vi "CosimModulator.vi"() -> ()   [LabVIEW 2017]
uses:
  FPGA/modInput.ctl
  <vilib>/Simulation/Scripting/Companion Diagram/SimConfigNode/SimParams.ctl
  <vilib>/Simulation/Scripting/Companion Diagram/SimConfigNode/_simSolvers.ctl
  <vilib>/Simulation/Implementation/Shared/SIMSCR Execution Mode.ctl
  <vilib>/Simulation/Param Hierarchy/Typedefs/SIMPH Param Control Actions.ctl
  <vilib>/Simulation/Implementation/Shared/NILVSim_ParamChanged.vi
  <vilib>/Simulation/Implementation/Shared/NILVSIM_BeginStep.vi
  <vilib>/Utility/error.llb/Clear Errors.vi
  <vilib>/rvi/Emulation/niFpgaSctlEmulationGetInTimedLoop.vi
  <vilib>/Simulation/Utility/Implementation/SIM Halt.vi
  <vilib>/Simulation/Implementation/Shared/NILVSim_Manager.vi
  <vilib>/Simulation/Implementation/Shared/NILVSim_FinalizeModel.vi
  <vilib>/Simulation/Implementation/Shared/SIM Unbundle Sim Info.vi
  <vilib>/Simulation/Implementation/Shared/NILVSim_Initialize.vi
  FPGA/Modulator.vi
  <vilib>/rvi/DataTransferAndStorage/Container/Common/niFpgaContainerExecOnDevCompGetState.vi
  <vilib>/rvi/Emulation/niFpgaEmulationIsFPGAContextNoSignature.vi
  <vilib>/rvi/DataTransferAndStorage/Container/Common/niFpgaContainerGetUniqueNameForEmu.vi
  <vilib>/rvi/Memory/Memory_Emulation/niFpgaMemoryEmulationCacheClearOnFirstRun.vi
  <vilib>/rvi/Memory/Memory_Emulation/nirvimemoryEmulationManagerCache_MakeExclusive.vi
  <vilib>/rvi/Memory/Memory_Emulation/niFpgaMemoryEmulationValidateCache.vi
  <vilib>/rvi/Memory/Memory_Emulation/nirvimemoryEmulationManagerCache_InsertValue.vi
  <vilib>/rvi/Memory/Memory_Emulation/nirvimemoryEmulationManagerCache_ReleaseExclusive.vi
  <vilib>/rvi/Memory/Memory_Emulation/nirvimemoryEmulationManagerCache_GetValue.vi
  <vilib>/rvi/Memory/Memory_Emulation/nirvimemoryEmulationManagerCache_SetValue.vi
  <vilib>/rvi/Emulation/niFpgaProcessEmulError.vi
  <vilib>/Simulation/Utility/Implementation/NILVSim Get Time and IsAcceptedStep.vi
  <vilib>/Simulation/Implementation/Shared/SIMSH Read Queue.vi
  <vilib>/Simulation/Implementation/Shared/NILVSim_GetModelError.vi
  <vilib>/Simulation/Implementation/Shared/SIM Bundle Sim Info.vi
  <vilib>/Simulation/Scripting/Companion Diagram/SimConfigNode/SimDog.xnode
  <vilib>/rvi/DataTransferAndStorage/Container/XNode/niFpgaContainer.xnode
  <vilib>/rvi/DataTransferAndStorage/Register/Emulation/niFpgaRegisterEmulationRefIn.vi
  <vilib>/Simulation/Implementation/XNodeFramework/SimXNode/SimX.xnode
  <vilib>/Simulation/EMI/Plugins/Multisim Design/MultisimEMICtrl.dll
  FPGA/BuckBoost.lvlib
  <vilib>/Simulation/Implementation/Shared/NI_SIM_Implementation.lvlib
panel:
  out "Data":u8 format="%.0x"
  in  "Disable":bool=TRUE
  in  "input":T1={"signal"=[0.5, 0.0, 0.0, 0.0]}
  out "Waveforms":dbl[][](graph)=[[-1.8615495247541, -18.191673880996113, -18.191673880996404, 8.184342820853757, 0.0, 1.0]]
  in  "Halt?":bool
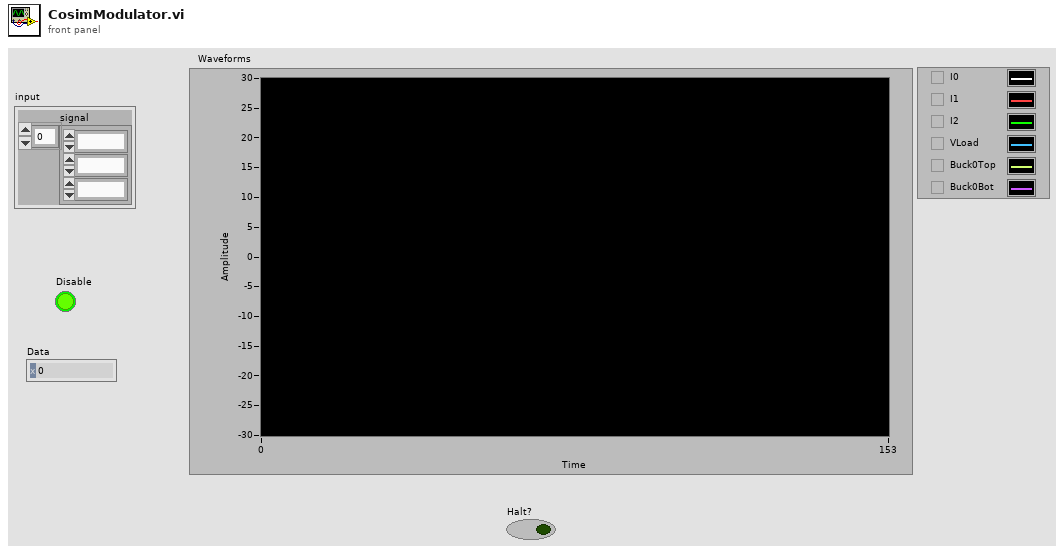
[diagram p1: front panel]
types:
  T1 = typedef "BuckBoost.lvlib/modInput.ctl" = cluster{"signal":fxp<+,18,0>[]}
  T2 = typedef "BuckBoost.lvlib/modRegisters.ctl" = cluster{"numberOfInterleaves":refnum<k21>, "Enable":refnum<k21>, "triangleInc":refnum<k21>, "Deadband":refnum<k21>, "Enabled":refnum<k21>}
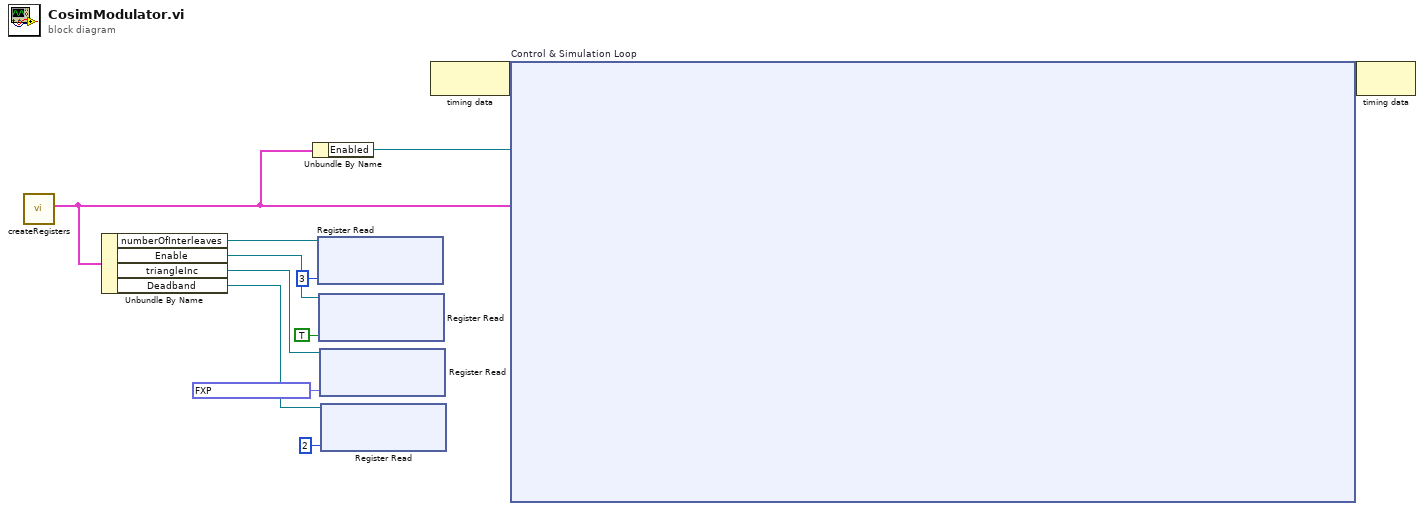
[diagram p0: block diagram]
diagram:
  n1 = call "createRegisters.vi"() -> ("modRegisters"=w2:T2)  [unwired: 10 in, 1 out]
  n2 = Unbundle By Name(w2) -> ("numberOfInterleaves"=w10:refnum<k21>, "Enable"=w9:refnum<k21>, "triangleInc"=w8:refnum<k21>, "Deadband"=w7:refnum<k21>)
  n3 = Unbundle By Name(w2) -> ("Enabled"=w1:refnum<k21>)
  n4 = xnode ("Register Read")("Data"=u8 3, "Register In"=w10) -> ()  [unwired: 1 out]
  n5 = xnode ("Register Read")("Data"=TRUE, "Register In"=w9) -> ()  [unwired: 1 out]
  n6 = xnode ("Register Read")("Data"=fxp<+,18,0> 0.09999847412109375, "Register In"=w8) -> ()  [unwired: 1 out]
  n7 = xnode ("Register Read")("Data"=u16 2, "Register In"=w7) -> ()  [unwired: 1 out]
  n8 = node-c288() -> (w12:variant)  [unwired: 1 in]
  n9 = node-c254 "Control & Simulation Loop"(w12, w2, w1) -> (w11:variant)
  n10 = node-c288(w11) -> ()  [unwired: 1 out]
